vi "Templating Service.vi"(8 "error in (no error)":errorcluster, 11 "Server in":refnum<class "Server.lvclass">) -> (0 "error out":errorcluster, 2 "Templating Service":refnum<class "TemplateService.lvclass">, 3 "Server out":refnum<class "Server.lvclass">)   [LabVIEW 2020, in "HTTP Server.lvlib" / "Server.lvclass"]
uses:
  Server.lvclass
  Server.lvclass/Server.ctl
  TemplateService/TemplateService.lvclass
  C:/dev/lv20CE/relink/lv-http-server/HTTP Server/TemplateService/TemplateService.lvclass
  C:/dev/lv20CE/relink/lv-http-server/HTTP Server/Service/Service.lvclass
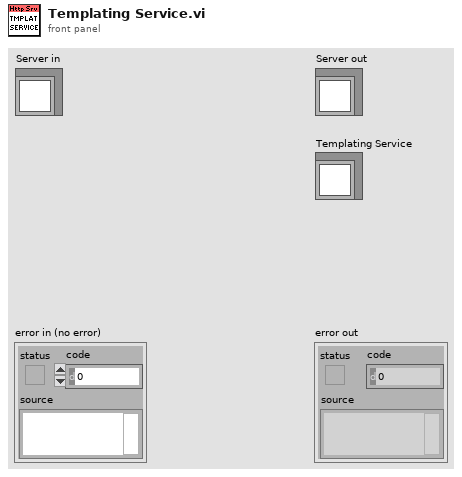
[diagram p1: front panel]
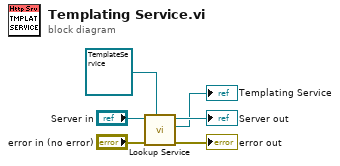
[diagram p0: block diagram]
diagram:
  n1 = call "Lookup Service.vi"("Service Type"=refnum<class "TemplateService.lvclass"> refnum ("HTTP Server:TemplateService.lvclass"), "error in (no error)"="error in (no error)", "Server in"="Server in") -> ("error out"=→"error out":errorcluster, "Service"=→"Templating Service":refnum<class "TemplateService.lvclass">, "Server out"=→"Server out":refnum<class "Server.lvclass">)  [unwired: 6 in]
